vi "LCD Control.vi"() -> ()   [LabVIEW 2025]
panel:
  in  "Cluster LCD":T1={"Direccion"=4, "Columna"=0, "Fila"=0, "Texto"=""} {"Fila" format="%x"; "Columna" format="%x"; "Direccion" min=4 max=40 format="%x"}
  out "error out":errorcluster
  out "read buffer":string
  in  "VISA resource name":refnum<visa-resource-name>
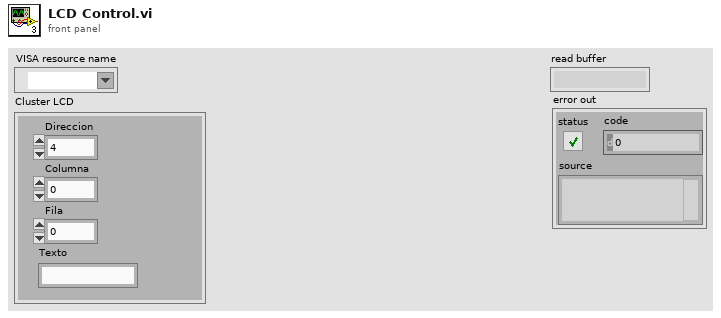
[diagram p1: front panel]
types:
  T1 = cluster{"Direccion":u8, "Columna":u8, "Fila":u8, "Texto":string}
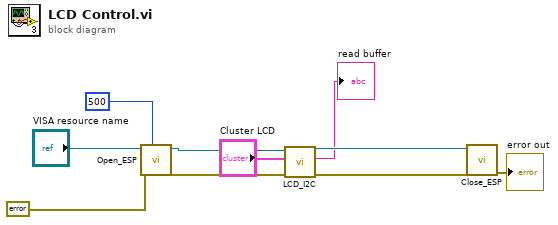
[diagram p0: block diagram]
diagram:
  n1 = call "Open_ESP.vi"("timeout (10sec)"=u32 500, "error in (no error)"=errorcluster {"status"=FALSE, "code"=0, "source"=""}, "VISA resource name"="VISA resource name") -> ("error out"=w6:errorcluster, "VISA resource name out"=w8:refnum<visa-resource-name>)  [unwired: 7 in]
  n2 = call "LCD_I2C.vi"("error in (no error)"=w6, "Cluster LCD"="Cluster LCD", "VISA resource name"=w8) -> ("error out"=w5:errorcluster, "read buffer"=→"read buffer":string, "VISA resource name out"=w4:refnum<visa-resource-name>)  [unwired: 6 in]
  n3 = call "Close_ESP.vi"("error in (no error)"=w5, "VISA resource name"=w4) -> ("error out"=→"error out":errorcluster)  [unwired: 9 in]
